vi "ReversedEngineering GetClassAttrubutes.vi"(1 "Path(CtrlRenumf used if Path is empty)":path, 2 "CtlRefnum":refnum<vi>, 5 "error in (no error)":errorcluster) -> (12 "LibraryName":string, 15 "attributeInfo":T1[](array[typedef]), 19 "error out":errorcluster)   [LabVIEW 2012]
uses:
  <resource>/Framework/Providers/Open_GDS/UML/ReversedEngineering/ReversedEngineering AttributeInfoType.ctl
  <resource>/Framework/Providers/Open_GDS/ClassProviders/Common/CommonVIs/CommonVIs_AttributeDataType.ctl
  <resource>/Framework/Providers/Open_GDS/UML/UMLEditor/UMLEditor_VisibilityType.ctl
  <resource>/Framework/Providers/Open_GDS/UML/UmlEditor_class/UmlEditor.lvclass
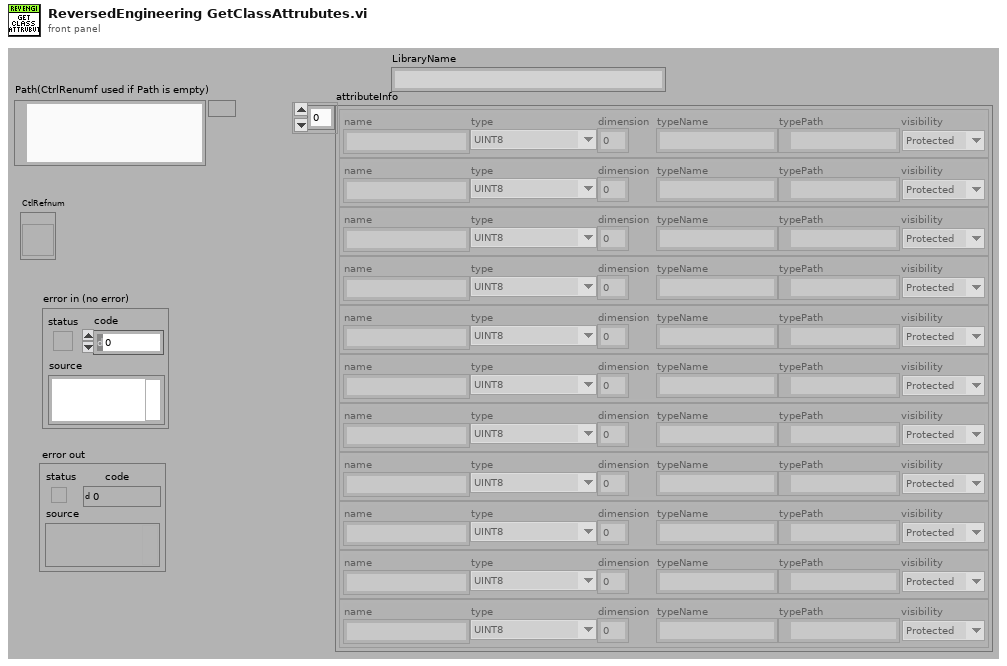
[diagram p1: front panel]
types:
  T1 = typedef "ReversedEngineering AttributeInfoType.ctl" = cluster{"name":string, "type":T2, "dimension":i32, "typeName":string, "typePath":path, "visibility":T3}
  T2 = typedef "CommonVIs_AttributeDataType.ctl" = enum16{"UINT8", "INT8", "UINT16", "INT16", "UINT32", "INT32", "UINT64", "INT64", "SGL", "DBL", "EXT", "CSG", "CDB", "CXT", "TimeStamp", "STRING", "PATH", "BOOL", "ENUM", "RefNum", "VIRefNum", "LabVIEW Class", "Cluster", "Variant", "TypeDef", "Waveform", "LabVIEW Object", "Other", "void"}
  T3 = typedef "UMLEditor_VisibilityType.ctl" = enum16{"Public", "Private", "Protected"}
  T4 = cluster{"name":string, "typeDesc":i16[], "dim":i32, "Path":string}[]
  T5 = cluster{"Label.Text":string, "Type DescriptorNonNameDependent":i16[], "index":i32, string}
  T6 = cluster{"Label.Text":string, "Type DescriptorNonNameDependent":i16[], "index":i32, "Path":string}[]
  T7 = cluster{"Label.Text":string, "typeDesc":i16[], "dim":i32, "Path":string}[]
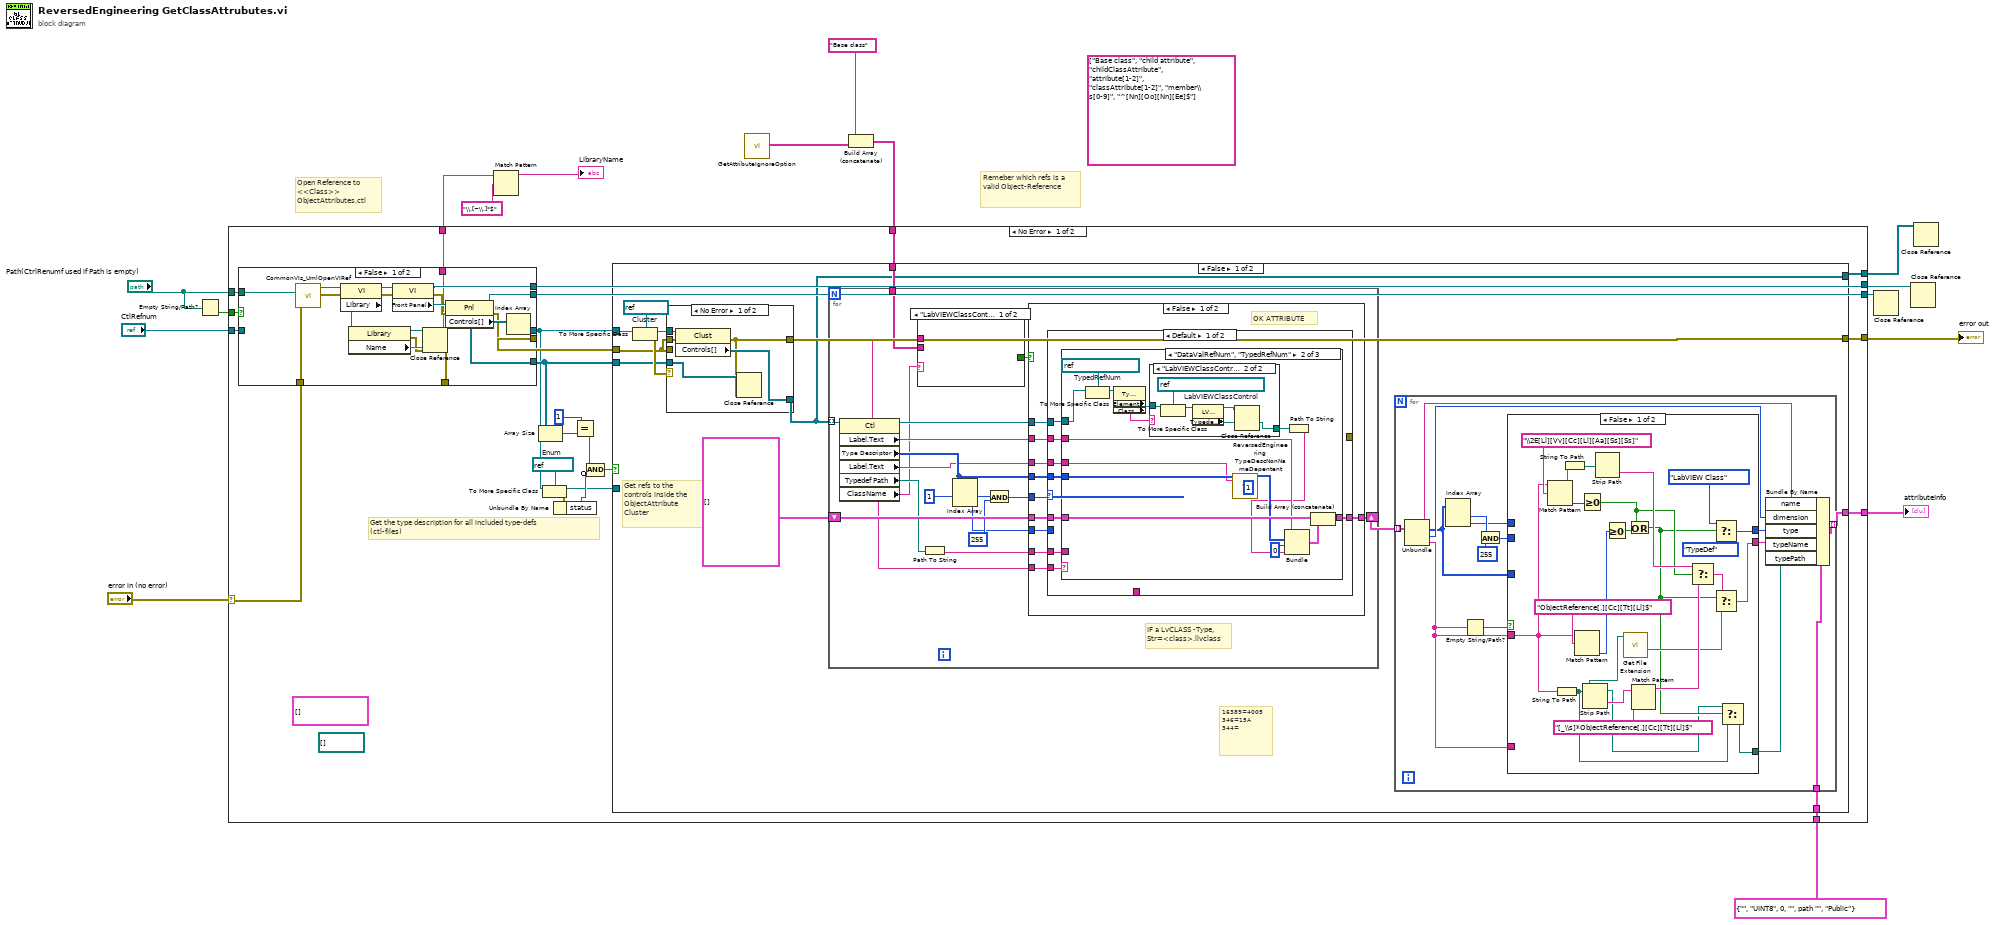
[diagram p0: block diagram]
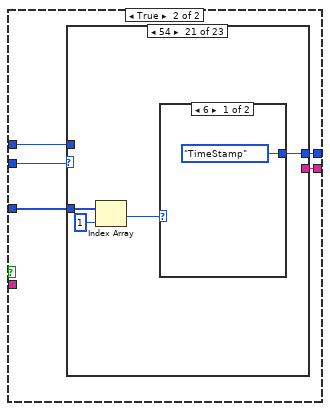
[diagram p3: hidden frame]
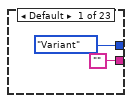
[diagram p4: hidden frame]
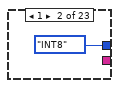
[diagram p5: hidden frame]
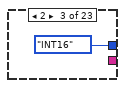
[diagram p6: hidden frame]
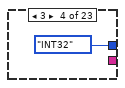
[diagram p7: hidden frame]
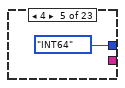
[diagram p8: hidden frame]
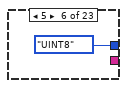
[diagram p9: hidden frame]
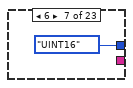
[diagram p10: hidden frame]
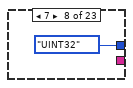
[diagram p11: hidden frame]
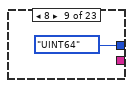
[diagram p12: hidden frame]
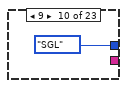
[diagram p13: hidden frame]
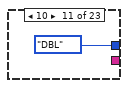
[diagram p14: hidden frame]
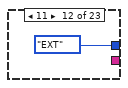
[diagram p15: hidden frame]
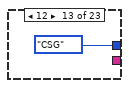
[diagram p16: hidden frame]
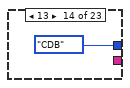
[diagram p17: hidden frame]
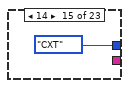
[diagram p18: hidden frame]
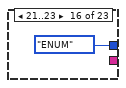
[diagram p19: hidden frame]
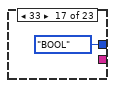
[diagram p20: hidden frame]
diagram:
  (unwired) string[] ["Base class", "child attribute", "childClassAttribute", "attribute[1-2]", "classAttribute[1-2]", "member\\s[0-9]", "^[Nn][Oo][Nn][Ee]$"]
  # "Remeber which refs is a valid Object-Reference"
  # "Open Reference to <<Class>> ObjectAttributes.ctl"
  n1 = Empty String/Path?(string/path="Path(CtrlRenumf used if Path is empty)") -> (empty?=w8:bool)
  n2 = call <resource>:"GetAttributeIgnoreOption.vi"() -> ("Attr"=w2:string[])  [unwired: 1 in, 18 out]
  n3 = Build Array (concatenate)("Base class", w2) -> (w1:string[])
  n4 = case shown="No Error" "error in (no error)" {
    selector: "error in (no error)" -> [w31 w271]
    tunnel: [w39 _] -> w16
    tunnel: [w38 w271] -> w11
    tunnel: [w37 _] -> w15
    tunnel: w1 -> [w36 _]
    tunnel: [w35 _] -> w14
    tunnel: T1 {"name"="", "type"=enum."UINT8", "dimension"=0, "typeName"="", "typePath"=path "", "visibility"=enum."Public"} ("attributeInfoType") -> [w34 _]
    tunnel: [w32 _] -> w12
    tunnel: "Path(CtrlRenumf used if Path is empty)" -> [w30 _]
    tunnel: w8 -> [w29 _]
    tunnel: "CtlRefnum" -> [w28 _]
    tunnel: [w17 _] -> w6
    frame No Error {
      w26 = refnum<vi> refnum  # Enum
      (unwired) path[] []
      (unwired) cluster{i16[]}[] []
      # "Get the type description for all included type-defs (ctl-files)"
      n5 = case shown="False" w29 {
        tunnel: [w264 w269] -> w25
        tunnel: [w262 _] -> w39
        tunnel: [w261 _] -> w35
        tunnel: [w260 w268] -> w27
        tunnel: [w259 w270] -> w33
        tunnel: w31 -> [w253 w270]
        tunnel: w30 -> [w256 _]
        tunnel: w28 -> [_ w269]
        tunnel: [w257 _] -> w17
        tunnel: [w250 _] -> _
        frame False {
          n6 = call <resource>:"CommonVIs_UmlOpenVIRef.vi"("error in"=w253, "ViPath/ViName"=w256) -> ("error out"=w255:errorcluster, "vi reference"=w254:refnum<vi>)  [unwired: 2 in, 6 out]
          n7 = property class="VI"(reference=w254, error in=w255) -> (reference out=w267:refnum<vi>, error out=w266:errorcluster, "Library"=w258:refnum<vi>)
          n8 = property class="Library"(reference=w258) -> (reference out=w252:refnum<vi>, error out=w251:errorcluster, "Name"=w257:string)  [unwired: 1 in]
          n9 = property class="VI"(reference=w267, error in=w266) -> (reference out=w262:refnum<vi>, error out=w263:errorcluster, "Front Panel"=w265:refnum<vi>)
          n10 = Close Reference(reference=w252, error in (no error)=w251) -> (error out=w250:errorcluster)
          n11 = property class="Pnl"(reference=w265, error in=w263) -> (reference out=w261:refnum<vi>, error out=w259:errorcluster, "Controls[]"=w260:refnum<vi>[])
          n12 = Index Array(array=w260) -> (element=w264:refnum<vi>)  [unwired: 1 in]
        }
        frame True {
          n13 = Build Array(w269) -> (w268:refnum<vi>[])
        }
      }
      n14 = Array Size(array=w27) -> (size(s)=w23:i32)
      n15 = To More Specific Class(target class=w26, reference=w25) -> (specific class reference=w18:refnum<vi>, error out=w24:errorcluster)  [unwired: 1 in]
      n16 = Unbundle By Name(w24) -> ("status"=w21:bool)
      n17 = Equal?(x=1, y=w23) -> (x = y?=w20:bool)
      n18 = Compound Arithmetic op=AND(w20, invert w21) -> (w19:bool)
      n19 = case shown="False" w19 {
        tunnel: [w50 w242] -> w38
        tunnel: [w47 w243] -> w37
        tunnel: w36 -> [w46 _]
        tunnel: w34 -> [w45 _]
        tunnel: w33 -> [w43 w241]
        tunnel: [w42 w240] -> w32
        tunnel: w27 -> [w41 w240]
        tunnel: w25 -> [w40 _]
        tunnel: w18 -> [_ w246]
        frame False {
          w52 = refnum<vi> refnum  # Cluster
          # "16389=4005\n346=15A\n344="
          # "Get refs to the controls inside the ObjectAttribute Cluster"
          n20 = To More Specific Class(target class=w52, reference=w40) -> (specific class reference=w51:refnum<vi>, error out=w44:errorcluster)  [unwired: 1 in]
          n21 = case shown="No Error" w44 {
            tunnel: w51 -> [w57 _]
            tunnel: [w55 w58] -> w42
            tunnel: w43 -> [w56 _]
            tunnel: [w53 w59] -> w50
            tunnel: w41 -> [w54 w58]
            tunnel: w43 -> [_ w59]
            frame No Error {
              n22 = property class="Clust"(reference=w57, error in=w56) -> (error out=w53:errorcluster, "Controls[]"=w55:refnum<vi>[])  [unwired: 1 out]
              n23 = Close Reference(reference=w54, error in (no error)=w53) -> ()  [unwired: 1 out]
            }
            frame Error {
            }
          }
          n24 = for {
            tunnel: w42 -> [w142] mode=indexing
            shift-right: [w151] -> w48
            shift-left: T4 [] -> [w152]
            tunnel: w46 -> [w143]
            # "IF a LvCLASS -Type,\nStr=<class>.llvclass"
            n25 = property class="Ctl"(reference=w142) -> (reference out=w137:refnum<vi>, "Label.Text"=w141:string, "Type Descriptor"=w146:i16[], "Label.Text"=w140:string, "Typedef Path"=w139:path, "ClassName"=w136:string)  [unwired: 1 in, 1 out]
            n26 = case shown="\"LabVIEWClassControl\"" w136 {
              tunnel: [_ w155] -> w144
              tunnel: w143 -> [_ w154]
              tunnel: w141 -> [_ w153]
              frame "LabVIEWClassControl" {
              }
              frame Default {
                n27 = for {
                  tunnel: [w159] -> w156 mode=indexing
                  tunnel: w153 -> [w158]
                  tunnel: w154 -> [w157] mode=indexing
                  n28 = Match Pattern(string=w158, regular expression=w157) -> (offset past match=w160:i32)  [unwired: 4 out]
                  n29 = Greater Or Equal To 0?(x=w160) -> (x >= 0?=w159:bool)
                }
                n30 = Or Array Elements(Boolean array=w156) -> (logical OR=w155:bool)
              }
            }
            n31 = Path To String(path=w139) -> (string=w138:string)
            n32 = Index Array(array=w146, index #1=1 ("index")) -> (element #1=w149:i16, element #2=w145:i16)  [unwired: 1 in]
            n33 = And(x=w149, y=i16 255) -> (x .and. y?=w147:i16)
            n34 = case shown="False" w144 {
              tunnel: w152 -> [w170 w239]
              tunnel: [w169 w239] -> w151
              tunnel: w147 -> [w168 _]
              tunnel: w146 -> [w167 _]
              tunnel: w145 -> [w166 _]
              tunnel: w141 -> [w165 _]
              tunnel: w140 -> [w164 _]
              tunnel: w138 -> [w163 _]
              tunnel: w137 -> [w162 _]
              tunnel: w136 -> [w161 _]
              frame False {
                # "OK ATTRIBUTE"
                n35 = case shown="Default" w168 {
                  tunnel: w170 -> [w178 w238]
                  tunnel: [w177 w237] -> w169
                  tunnel: w167 -> [w175 w232]
                  tunnel: w166 -> [_ w228]
                  tunnel: w165 -> [w176 w226]
                  tunnel: w164 -> [w174 _]
                  tunnel: w163 -> [w173 _]
                  tunnel: w162 -> [w171 w224]
                  tunnel: [_ w218] -> _
                  tunnel: [_ w217] -> _
                  tunnel: w161 -> [w172 _]
                  frame Default {
                    n36 = case shown="\"DataValRefNum\", \"TypedRefNum\"" w172 {
                      tunnel: w178 -> [w187 w202 w216]
                      tunnel: [w186 w201 w215] -> w177
                      tunnel: w176 -> [w184 w199 w213]
                      tunnel: w175 -> [w182 w197 w211]
                      tunnel: w174 -> [w181 w196 w210]
                      tunnel: w173 -> [w179 _ w208]
                      tunnel: w171 -> [_ w190 _]
                      frame Default {
                        (unwired) 1 ("index")
                        n37 = call <resource>:"ReversedEngineering TypeDescNonNameDepentent.vi"("Type DescriptorNameDependent"=w182, "LabelText"=w181) -> ("Type DescriptorNonNameDependent"=w180:i16[])  [unwired: 17 out]
                        n38 = Bundle("Label.Text"=w184, "Type DescriptorNonNameDependent"=w180, "index"=0, w179) -> (w185:T5)  [unwired: 1 out]
                        n39 = Build Array (concatenate)(w187, w185) -> (w186:T6)
                      }
                      frame "DataValRefNum", "TypedRefNum" {
                        w194 = refnum<vi> refnum  # TypedRefNum
                        (unwired) 1 ("index")
                        n40 = To More Specific Class(target class=w194, reference=w190) -> (specific class reference=w193:refnum<vi>)  [unwired: 1 in, 1 out]
                        n41 = property class="TypRef"(reference=w193) -> ("Element"=w191:refnum<vi>, "Element.ClassName"=w192:string)  [unwired: 1 in, 2 out]
                        n42 = case shown="\"LabVIEWClassControl\"" w192 {
                          tunnel: w191 -> [_ w206]
                          tunnel: [_ w204] -> w189
                          frame "False", Default {
                          }
                          frame "LabVIEWClassControl" {
                            w207 = refnum<vi> refnum  # LabVIEWClassControl
                            n43 = To More Specific Class(target class=w207, reference=w206) -> (specific class reference=w205:refnum<vi>)  [unwired: 1 in, 1 out]
                            n44 = property class="LVClassControl"(reference=w205) -> (reference out=w203:refnum<vi>, "Typedef Path"=w204:path)  [unwired: 1 in, 1 out]
                            n45 = Close Reference(reference=w203) -> ()  [unwired: 1 in, 1 out]
                          }
                        }
                        n46 = call <resource>:"ReversedEngineering TypeDescNonNameDepentent.vi"("Type DescriptorNameDependent"=w197, "LabelText"=w196) -> ("Type DescriptorNonNameDependent"=w195:i16[])  [unwired: 17 out]
                        n47 = Path To String(path=w189) -> (string=w188:string)
                        n48 = Bundle("Label.Text"=w199, "Type DescriptorNonNameDependent"=w195, "index"=0, w188) -> (w200:T5)  [unwired: 1 out]
                        n49 = Build Array (concatenate)(w202, w200) -> (w201:T6)
                      }
                      frame "LabVIEWClassControl" {
                        (unwired) 1 ("index")
                        n50 = call <resource>:"ReversedEngineering TypeDescNonNameDepentent.vi"("Type DescriptorNameDependent"=w211, "LabelText"=w210) -> ("Type DescriptorNonNameDependent"=w209:i16[])  [unwired: 17 out]
                        n51 = Bundle("Label.Text"=w213, "Type DescriptorNonNameDependent"=w209, "index"=0, w208) -> (w214:T5)  [unwired: 1 out]
                        n52 = Build Array (concatenate)(w216, w214) -> (w215:T6)
                      }
                    }
                  }
                  frame 64 {
                    w223 = refnum<vi> refnum  # Array
                    n53 = To More Specific Class(target class=w223, reference=w224) -> (specific class reference=w222:refnum<vi>, error out=w219:errorcluster)  [unwired: 1 in]
                    n54 = property class="Arr"(reference=w222, error in=w219) -> (error out=w218:errorcluster, "Array Element.Typedef Path"=w221:path, "ClassName"=w217:string)  [unwired: 1 out]
                    n55 = Path To String(path=w221) -> (string=w220:string)
                    n56 = Multiply(x=w228, y=i16 2) -> (x*y=w235:i16)
                    n57 = Search 1D Array(1D array=w232, element=i16 25856) -> (index of element=w231:i32)  [unwired: 1 out]
                    n58 = Increment(x=w231) -> (x+1=w229:i32)
                    n59 = Add(x=w235, y=i16 4) -> (x+y=w230:i16)
                    n60 = Subtract(x=w229, y=w230) -> ()  [unwired: 1 out]
                    n61 = Array Subset(array=w232, index=w230) -> (w227:i16[])  [unwired: 1 in]
                    n62 = Bundle("Label.Text"=w226, w227, w228, w220) -> (w225:cluster{"Label.Text":string, i16[], i16, string})  [unwired: 1 out]
                    n63 = Build Array (concatenate)(w238, w225) -> (w237:T7)
                  }
                }
              }
              frame True {
                # "IGNORE SINCE IT IS A DEFAULT\nATTRIBUTE THAT HAS TO EXIST"
              }
            }
          }
          n64 = for {
            tunnel: w48 -> [w74] mode=indexing
            tunnel: w45 -> [w70]
            tunnel: [w65] -> w47 mode=indexing
            n65 = Unbundle(w74) -> ("name"=w69:string, "typeDesc"=w64:i16[], "dim"=w68:i32, "Path"=w62:string)
            n66 = Index Array(array=w64) -> (element #1=w72:i16, element #2=w60:i16)  [unwired: 2 in]
            n67 = Empty String/Path?(string/path=w62) -> (empty?=w63:bool)
            n68 = And(x=w72, y=i16 255) -> (x .and. y?=w71:i16)
            n69 = case shown="False" w63 {
              tunnel: w71 -> [_ w102]
              tunnel: [w95 w101] -> w67
              tunnel: [w91 w100] -> w66
              tunnel: w64 -> [_ w99]
              tunnel: w62 -> [w83 _]
              tunnel: w62 -> [_ _]
              tunnel: [w76 _] -> w61
              tunnel: w60 -> [_ w98]
              frame False {
                n70 = Match Pattern(string=w83, regular expression="\\2E[Ll][Vv][Cc][Ll][Aa][Ss][Ss]") -> (before substring=w85:string, offset past match=w88:i32)  [unwired: 3 out]
                n71 = String To Path(string=w83) -> (path=w75:path)
                n72 = String To Path(string=w85) -> (path=w84:path)
                n73 = Match Pattern(string=w83, regular expression="ObjectReference[.][Cc][Tt][Ll]$") -> (offset past match=w93:i32)  [unwired: 4 out]
                n74 = Greater Or Equal To 0?(x=w88) -> (x >= 0?=w80:bool)
                n75 = Strip Path(path=w75) -> (stripped path=w77:path, name=w90:string)
                n76 = Strip Path(path=w84) -> (name=w82:string)  [unwired: 1 out]
                n77 = Greater Or Equal To 0?(x=w93) -> (x >= 0?=w92:bool)
                n78 = call <vilib>:"Get File Extension.vi"("file"=w75) -> ("filename without extension"=w79:string)  [unwired: 1 in, 9 out]
                n79 = Or(x=w80, y=w92) -> (x .or. y?=w78:bool)
                n80 = Match Pattern(string=w90, regular expression="[_\\s]*ObjectReference[.][Cc][Tt][Ll]$") -> (before substring=w86:string)  [unwired: 4 out]
                n81 = Select(t=w82, s=w80, f=w86) -> (s? t:f=w87:string)
                n82 = Select(t=CommonVIs_AttributeDataType."LabVIEW Class" ("type"), s=w78, f=CommonVIs_AttributeDataType."TypeDef" ("type")) -> (s? t:f=w95:T2)
                n83 = Select(t=w87, s=w78, f=w79) -> (s? t:f=w91:string)
                n84 = Select(t=w77, s=w78, f=w75) -> (s? t:f=w76:path)
              }
              frame True {
                n85 = case shown="54" w102 {
                  tunnel: w99 -> [_ _ _ _ _ _ _ _ _ _ _ _ _ _ _ _ _ _ _ _ w126 _ _]
                  tunnel: [CommonVIs_AttributeDataType."Variant" ("type") CommonVIs_AttributeDataType."INT8" ("type") CommonVIs_AttributeDataType."INT16" ("type") CommonVIs_AttributeDataType."INT32" ("type") CommonVIs_AttributeDataType."INT64" ("type") CommonVIs_AttributeDataType."UINT8" ("type") CommonVIs_AttributeDataType."UINT16" ("type") CommonVIs_AttributeDataType."UINT32" ("type") CommonVIs_AttributeDataType."UINT64" ("type") CommonVIs_AttributeDataType."SGL" ("type") CommonVIs_AttributeDataType."DBL" ("type") CommonVIs_AttributeDataType."EXT" ("type") CommonVIs_AttributeDataType."CSG" ("type") CommonVIs_AttributeDataType."CDB" ("type") CommonVIs_AttributeDataType."CXT" ("type") CommonVIs_AttributeDataType."ENUM" ("type") CommonVIs_AttributeDataType."BOOL" ("type") CommonVIs_AttributeDataType."STRING" ("type") CommonVIs_AttributeDataType."PATH" ("type") CommonVIs_AttributeDataType."Variant" ("type") w127 CommonVIs_AttributeDataType."Cluster" ("type") w133] -> w101
                  tunnel: ["" _ _ _ _ _ _ _ _ _ _ _ _ _ _ _ _ _ _ _ _ _ "" ("f")] -> w100
                  tunnel: w98 -> [_ _ _ _ _ _ _ _ _ _ _ _ _ _ _ _ _ _ _ _ _ _ w131]
                  frame Default {
                  }
                  frame 1 {
                  }
                  frame 2 {
                  }
                  frame 3 {
                  }
                  frame 4 {
                  }
                  frame 5 {
                  }
                  frame 6 {
                  }
                  frame 7 {
                  }
                  frame 8 {
                  }
                  frame 9 {
                  }
                  frame 10 {
                  }
                  frame 11 {
                  }
                  frame 12 {
                  }
                  frame 13 {
                  }
                  frame 14 {
                  }
                  frame 21..23 {
                  }
                  frame 33 {
                  }
                  frame 48 {
                  }
                  frame 50 {
                  }
                  frame 83 {
                  }
                  frame 84 {
                    n86 = Index Array(array=w126, index=1) -> (element=w124:i16)
                    n87 = case shown="6" w124 {
                      tunnel: [CommonVIs_AttributeDataType."TimeStamp" ("type") CommonVIs_AttributeDataType."Waveform" ("type")] -> w127
                      frame 6 {
                      }
                      frame Default {
                      }
                    }
                  }
                  frame 80 {
                    # "Cluster"
                  }
                  frame 112 {
                    # "RefNum"
                    n88 = case shown="30" w131 {
                      tunnel: [CommonVIs_AttributeDataType."RefNum" ("type") CommonVIs_AttributeDataType."LabVIEW Object" ("type")] -> w133
                      frame Default {
                      }
                      frame 30 {
                      }
                    }
                  }
                }
              }
            }
            n89 = Bundle By Name(cluster=w70, "name"=w69, "dimension"=w68, "type"=w67, "typeName"=w66, "typePath"=w61) -> (w65:T1)
          }
        }
        frame True {
          n90 = property class="Enum"(reference=w246, error in=w241) -> (error out=w242:errorcluster, "Strings []"=w244:string[])  [unwired: 1 out]
          n91 = for {
            tunnel: T1 {"name"="Enum", "type"=enum."Other", "dimension"=0, "typeName"="", "typePath"=path "", "visibility"=enum."Public"} ("attributeInfoType") -> [w249]
            tunnel: w244 -> [w248] mode=indexing
            tunnel: [w247] -> w243 mode=indexing
            n92 = Bundle By Name(cluster=w249, "name"=w248) -> (w247:T1)
          }
        }
      }
    }
    frame Error {
    }
  }
  "error out" <- w11
  "attributeInfo" <- w15
  n93 = Match Pattern(string=w6, regular expression="\\.[~\\.]*$") -> (before substring=→"LibraryName":string)  [unwired: 4 out]
  n94 = Close Reference(reference=w14) -> ()  [unwired: 1 in, 1 out]
  n95 = Close Reference(reference=w16) -> ()  [unwired: 1 in, 1 out]
  n96 = Close Reference(reference=w12) -> ()  [unwired: 1 in, 1 out]
